vi "Run Tests - When Test Passes - Sets Outcome To Passed.vi"() -> ()   [LabVIEW 2017, in "LVUnit Test Executor.Tests.lvlib"]
uses:
  LVUnit Test Executor.Tests.lvlib
  LVUnit Test Executor/LVUnit Test Executor.lvclass
  Test Outcome.ctl
  LVUnit Test Case/LVUnit Test Case.lvclass
  C:/Users/pasca/Projects/Home/lvunit/Test Case/Test Case.lvclass
  Test Result/Test Result.lvclass/Test Result.ctl
  Test Result/Get Outcome.vi
  Fake Passing Test.vi
  Test Case/Test Case.lvclass
  Test Result/Test Result.lvclass
  <vilib>/PNR/Transparent Assertions/Transparent Assertions/Transparent Assertions.lvlib
panel:
  out "error out":errorcluster
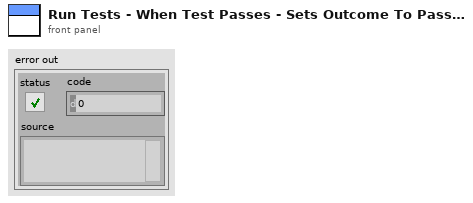
[diagram p1: front panel]
types:
  T1 = typedef "Test Outcome.ctl" = enum16{"None", "Passed", "Failed"}
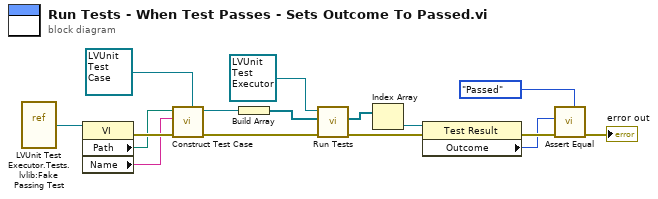
[diagram p0: block diagram]
diagram:
  n1 = vi-ref "LVUnit Test Executor.Tests.lvlib:Fake Passing Test.vi"() -> (w13:refnum<vi>)
  n2 = property class="VI"(reference=w13) -> (error out=w12:errorcluster, "Path"=w11:path, "Name"=w10:string)  [unwired: 1 in, 1 out]
  n3 = call "Construct Test Case.vi"("Test Case in"=refnum<class "LVUnit Test Case.lvclass"> refnum ("LVUnit Test Case"), "error in (no error)"=w12, "Qualified Name"=w10, "Path"=w11) -> ("error out"=w9:errorcluster, "Test Case out"=w8:refnum<class "LVUnit Test Case.lvclass">)  [unwired: 6 in]
  n4 = Build Array(w8) -> (w7:refnum<class "LVUnit Test Case.lvclass">[])
  n5 = call-dynamic "Run Tests.vi"("error in (no error)"=w9, "Test Cases"=w7, "LVUnit Test Executor in"=refnum<class "LVUnit Test Executor.lvclass"> refnum ("LVUnit Test Executor")) -> ("error out"=w15:errorcluster, "Test Results"=w5:refnum<class "Test Result.lvclass">[])  [unwired: 6 in, 1 out]
  n6 = Index Array(array=w5) -> (element=w4:refnum<class "Test Result.lvclass">)  [unwired: 1 in]
  n7 = property class="Test Result"(reference=w4, error in=w15) -> (error out=w6:errorcluster, "Outcome"=w3:T1)  [unwired: 1 out]
  n8 = call <vilib>:"Assert Equal.vi"("Expected"=Test_Outcome."Passed" ("Outcome"), "error in (no error)"=w6, "Actual"=w3) -> ("error out"=→"error out":errorcluster)  [unwired: 8 in]
